vi "isRefValid.vi"(8 "error in (no error)":errorcluster, 11 "xwpfDocument.Element in":refnum<class "xwpfDocument.Element.lvclass">) -> (0 "error out":errorcluster, 3 "xwpfDocument.Element out":refnum<class "xwpfDocument.Element.lvclass">)   [LabVIEW 2017, in "Word_Specific.lvlib" / "xwpfDocument.Element.lvclass"]
uses:
  xwpfDocument.Element.lvclass
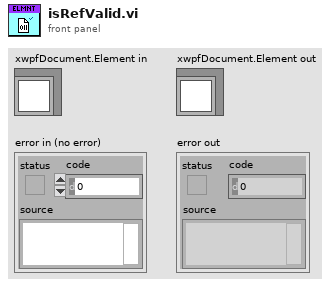
[diagram p1: front panel]
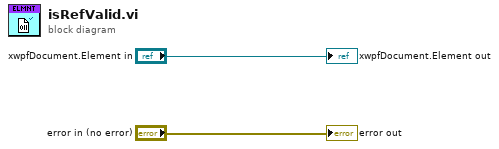
[diagram p0: block diagram]
diagram:
  "error out" <- "error in (no error)"
  "xwpfDocument.Element out" <- "xwpfDocument.Element in"
